vi "Create Test Configuration.vi"() -> (0 "error out":errorcluster, 1 "Names":string[](array[string]), 2 "Line Array":T1(array[cluster]), 3 "Module":refnum<class "ThreePhasePLL configuration.lvclass">, 4 "Channels":refnum<class "TBM channel.lvclass">[](array[class]), 5 "instance identifier":string)   [LabVIEW 2017, in "ThreePhasePLL tests.lvlib"]
uses:
  ThreePhasePLL tests.lvlib
  <vilib>/NI/Tag Bus Module Framework/channel/TBM channel.lvclass
  module/configuration/ThreePhasePLL configuration.lvclass
  C:/Program Files (x86)/National Instruments/LabVIEW 2017/vi.lib/NI/Configuration Framework/serializable configuration/NISE_CEF_serializable configuration.lvclass
  C:/Program Files (x86)/National Instruments/LabVIEW 2017/vi.lib/NI/DCAF/Tag Editor Core/control module/configuration/control module configuration.lvclass
  <vilib>/NI/Tag Bus Module Framework/channel/channel classification.ctl
  <vilib>/NI/Tag Bus/tag/Data Type.ctl
  <vilib>/NI/Configuration Framework/serializable configuration/NISE_CEF_serializable configuration.lvclass
  <vilib>/NI/Tag Bus/tag/tag descriptor.lvclass
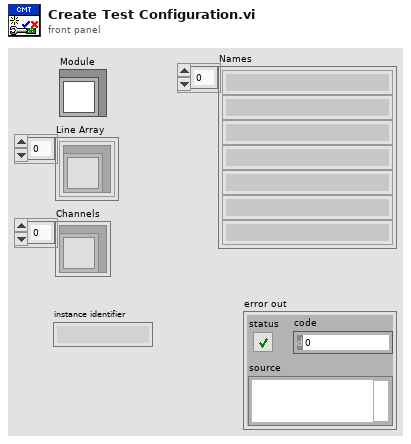
[diagram p1: front panel]
types:
  T1 = cluster{"channel":refnum<class "TBM channel.lvclass">}[]
  T2 = typedef "tag bus.lvlib/tag descriptor.lvclass/Data Type.ctl" = enum16{"Double", "Single", "I64", "I32", "I16", "I8", "U64", "U32", "U16", "U8", "Boolean", "String", "Array of Double", "Array of Single", "Array of I64", "Array of I32", "Array of I16", "Array of I8", "Array of U64", "Array of U32", "Array of U16", "Array of U8", "Array of Boolean", "Array of String"}
  T3 = typedef "TBM channel.lvclass/channel classification.ctl" = enum16{"input data", "output data", "processing parameter", "processing result"}
  T4 = cluster{"channel":refnum<class "TBM channel.lvclass">}
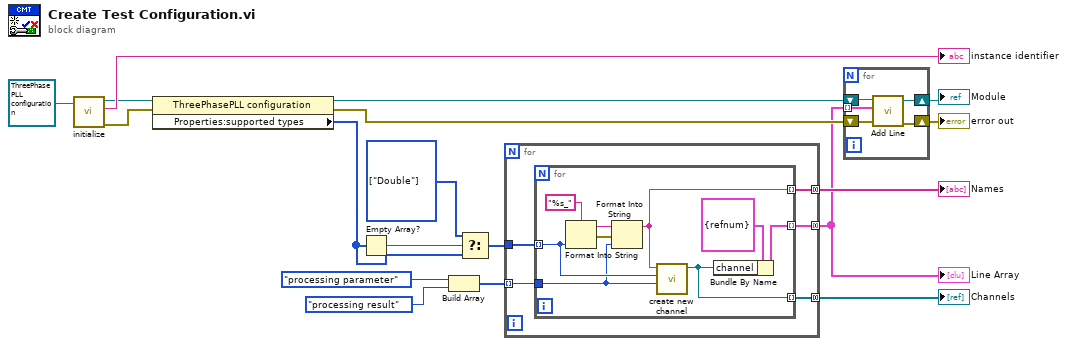
[diagram p0: block diagram]
diagram:
  w5 = T2[] [enum."Double"] items=["Double", "Single", "I64", "I32", "I16", "I8", "U64", "U32", "U16", "U8", "Boolean", "String", "Array of Double", "Array of Single", "Array of I64", "Array of I32", "Array of I16", "Array of I8", "Array of U64", "Array of U32", "Array of U16", "Array of U8", "Array of Boolean", "Array of String"] ("Properties:supported types")
  n1 = call <vilib>:"initialize.vi"("configuration in"=refnum<class "ThreePhasePLL configuration.lvclass"> refnum ("user control module configuration")) -> ("error out"=w17:errorcluster, "identifier"=→"instance identifier":string, "configuration out"=w14:refnum<class "ThreePhasePLL configuration.lvclass">)  [unwired: 8 in]
  n2 = property class="ThreePhasePLL configuration"(reference=w14, error in=w17) -> (reference out=w12:refnum<class "ThreePhasePLL configuration.lvclass">, error out=w16:errorcluster, "Properties:supported types"=w3:T2[])
  n3 = Empty Array?(array=w3) -> (empty?=w6:bool)
  n4 = Build Array(channel_classification."processing parameter" ("channel classification"), channel_classification."processing result" ("channel classification")) -> (w11:T3[])
  n5 = Select(t=w5, s=w6, f=w3) -> (s? t:f=w4:T2[])
  n6 = for {
    tunnel: w11 -> [w23] mode=indexing
    tunnel: [w21] -> w13 mode=concatenating
    tunnel: w4 -> [w22]
    tunnel: [w20] -> w15 mode=concatenating
    tunnel: [w19] -> w1 mode=concatenating
    n7 = for {
      tunnel: w23 -> [w27]
      tunnel: [w32] -> w21 mode=indexing
      tunnel: w22 -> [w29] mode=indexing
      tunnel: [w24] -> w20 mode=indexing
      tunnel: [w31] -> w19 mode=indexing
      n8 = Format Into String(format string="%s_", w29) -> (resulting string=w26:string, error out=w28:errorcluster)  [unwired: 2 in]
      n9 = Format Into String(initial string=w26, error in=w28, w27) -> (resulting string=w24:string)  [unwired: 1 in, 1 out]
      n10 = call <vilib>:"create new channel.vi"("channel classification"=w27, "data type"=w29, "channel name"=w24) -> ("channel"=w31:refnum<class "TBM channel.lvclass">)  [unwired: 8 in]
      n11 = Bundle By Name(cluster=T4 {"channel"=refnum} ("Line"), "channel"=w31) -> (w32:T4)
    }
  }
  "Names" <- w15
  "Channels" <- w1
  "Line Array" <- w13
  n12 = for {
    tunnel: w13 -> [w35] mode=indexing
    shift-right: [w36] -> w2
    shift-left: w12 -> [w37]
    shift-right: [w33] -> w7
    shift-left: w16 -> [w34]
    n13 = call-dynamic "Add Line.vi"("error in (no error)"=w34, "Line"=w35, "ThreePhasePLL configuration in"=w37) -> ("error out"=w33:errorcluster, "ThreePhasePLL configuration out"=w36:refnum<class "ThreePhasePLL configuration.lvclass">)  [unwired: 7 in]
  }
  "Module" <- w2
  "error out" <- w7
